vi "make PLL params.vi"(7 "self":enum16{"Diode", "RF mixer", "lockin"}(ring), 9 "scope settings":T1, 11 "PLL params in":T3={"f21 (kHz)"=20.0, "f43 (kHz)"=32.0, "f32 (kHz)"=47.0, "P gain"=2000.0, "I gain"=5.0, "LP BW (kHz)"=5.0, "notch BW (kHz)"=2.0}) -> (3 "param PLL2":T2)   [LabVIEW 2018]
uses:
  PLL param interface.ctl
  scope settings.ctl
  <vilib>/rvi/Analysis/host/Butterworth/config/Butterworth Filter Order.ctl
  <vilib>/rvi/Analysis/host/Butterworth/config/Butterworth Filter Type.ctl
  <vilib>/Analysis/polynomials.llb/Unique Numbers and Multiplicity (DBL).vi
  <vilib>/rvi/Analysis/host/Notch/config/NotchScaledCoefficients.vi
  <vilib>/rvi/Analysis/host/Butterworth/config/BwScaledCoefficients.vi
  <vilib>/rvi/Analysis/host/Notch/XNode/NotchCoefficients.xnode
  <vilib>/rvi/Analysis/host/Butterworth/XNode/ButterworthCoefficients.xnode
  <vilib>/rvi/Analysis/host/Public/NI_FpgaMspHost.lvlib
  <vilib>/Analysis/NI_AALPro.lvlib
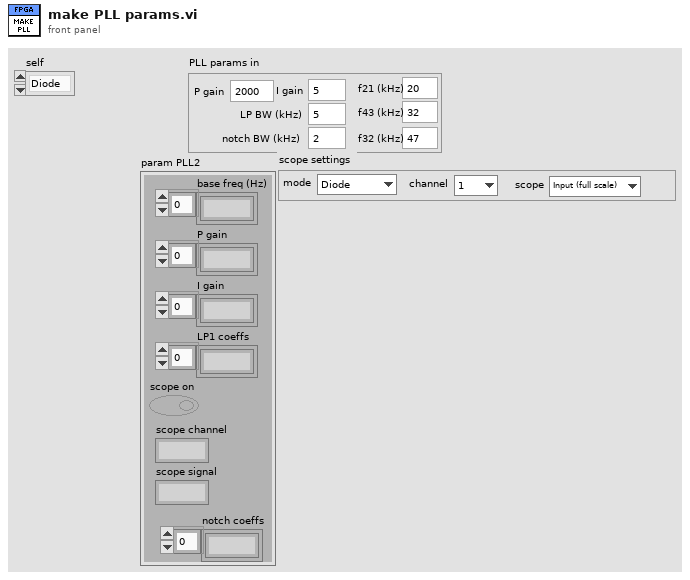
[diagram p1: front panel]
types:
  T1 = typedef "scope settings.ctl" = cluster{"mode":enum16{"Diode", "RF mixer", "lockin"}, "channel":enum16{"1", "2", "3"}, "scope":enum16{"Input (full scale)", "PLL out", "Phase error (deg)", "Freq. error (Hz)"}}
  T2 = cluster{"base freq (Hz)":fxp<+,17,17>[], "P gain":fxp<+,14,14>[], "I gain":fxp<+,20,6>[], "LP1 coeffs":i32[], "scope on":bool, "scope channel":u8, "scope signal":u8, "notch coeffs":i32[]}
  T3 = typedef "PLL param interface.ctl" = cluster{"f21 (kHz)":dbl, "f43 (kHz)":dbl, "f32 (kHz)":dbl, "P gain":dbl, "I gain":dbl, "LP BW (kHz)":dbl, "notch BW (kHz)":dbl}
  T4 = enum16{"Input (full scale)", "PLL out", "Phase error (deg)", "Freq. error (Hz)"}
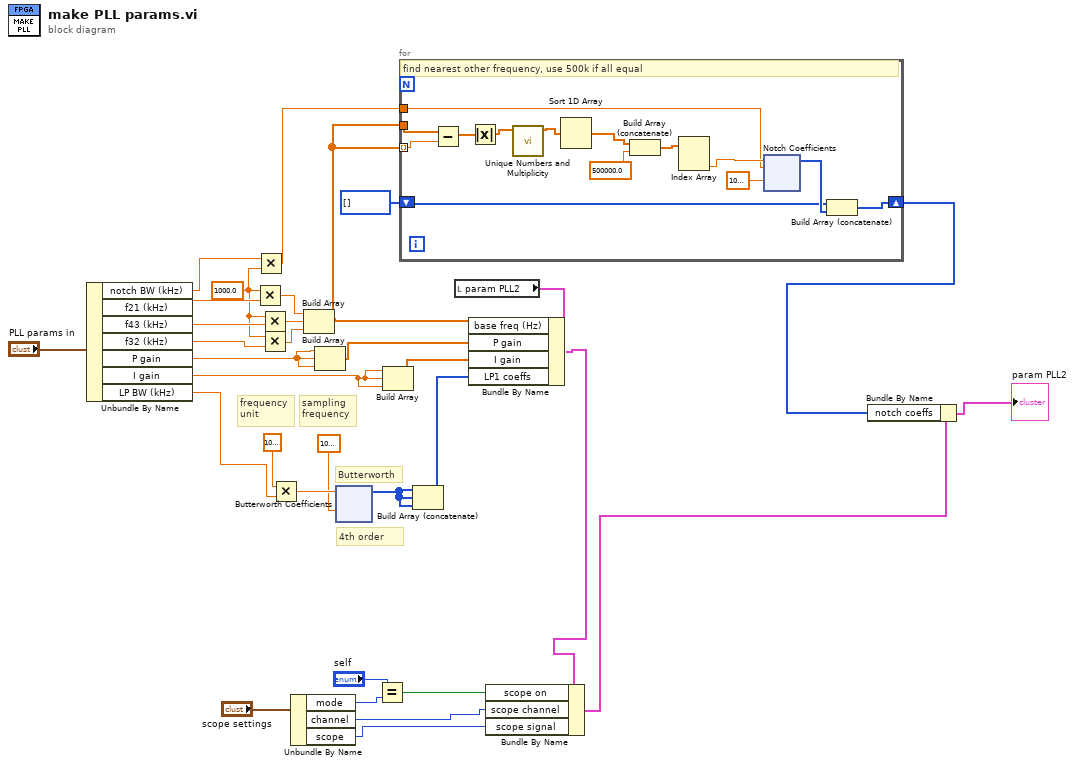
[diagram p0: block diagram]
diagram:
  w7 = 1000.0 ("x")
  # "4th order"
  # "Butterworth"
  # "frequency\nunit"
  # "sampling\nfrequency"
  n1 = Unbundle By Name("PLL params in") -> ("notch BW (kHz)"=w6:dbl, "f21 (kHz)"=w32:dbl, "f43 (kHz)"=w31:dbl, "f32 (kHz)"=w30:dbl, "P gain"=w26:dbl, "I gain"=w24:dbl, "LP BW (kHz)"=w19:dbl)
  n2 = Multiply(x=w7, y=w32) -> (x*y=w29:dbl)
  n3 = Multiply(x=w6, y=w7) -> (x*y=w5:dbl)
  n4 = Multiply(x=w7, y=w31) -> (x*y=w28:dbl)
  n5 = Multiply(x=w7, y=w30) -> (x*y=w27:dbl)
  n6 = Multiply(x=1000.0 ("sample rate (S/s)"), y=w19) -> (x*y=w22:dbl)
  n7 = Unbundle By Name("scope settings") -> ("mode"=w14:enum16{"Diode", "RF mixer", "lockin"}, "channel"=w10:enum16{"1", "2", "3"}, "scope"=w9:T4)
  n8 = Build Array(w29, w28, w27) -> (w8:dbl[])
  n9 = Build Array(w26, w26, w26) -> (w25:dbl[])
  n10 = xnode "Butterworth Coefficients"("cutoff frequency (Hz)"=w22, "sample rate (S/s)"=1000000.0) -> ("scaled coefficients"=w18:i32[])  [unwired: 1 in, 1 out]
  n11 = Equal?(x="self", y=w14) -> (x = y?=w11:bool)
  n12 = Build Array(w24, w24, w24) -> (w23:dbl[])
  n13 = for {
    tunnel: w8 -> [w47] mode=indexing
    tunnel: w8 -> [w46]
    tunnel: w5 -> [w37]
    shift-right: [w35] -> w2
    shift-left: i32[] [] -> [w34]
    # "find nearest other frequency, use 500k if all equal"
    n14 = Subtract(x=w46, y=w47) -> (x-y=w45:dbl[])
    n15 = Absolute Value(x=w45) -> (abs(x)=w44:dbl[])
    n16 = call-poly <vilib>:"Unique Numbers and Multiplicity.vi"("Numbers"=w44) -> ("Unique Numbers"=w43:dbl[])  [unwired: 8 in, 2 out]
    n17 = Sort 1D Array(array=w43) -> (sorted array=w42:dbl[])
    n18 = Build Array (concatenate)(w42, 500000.0) -> (w40:dbl[])
    n19 = Index Array(array=w40) -> (element #2=w39:dbl)  [unwired: 2 in, 1 out]
    n20 = xnode "Notch Coefficients"("notch frequency (Hz)"=w39, "notch width (Hz)"=w37, "sample rate (S/s)"=1000000.0) -> ("scaled coefficients"=w36:i32[])  [unwired: 1 in, 1 out]
    n21 = Build Array (concatenate)(w34, w36) -> (w35:i32[])
  }
  n22 = Build Array (concatenate)(w18, w18, w18) -> (w17:i32[])
  n23 = local read "param PLL2"() -> (w16:T2)
  n24 = Bundle By Name(cluster=w16, "base freq (Hz)"=w8, "P gain"=w25, "I gain"=w23, "LP1 coeffs"=w17) -> (w12:T2)
  n25 = Bundle By Name(cluster=w12, "scope on"=w11, "scope channel"=w10, "scope signal"=w9) -> (w3:T2)
  n26 = Bundle By Name(cluster=w3, "notch coeffs"=w2) -> (→"param PLL2":T2)
